vi "GUI.vi"() -> ()   [LabVIEW 2013]
uses:
  <vilib>/Instr/_visa.llb/VISA Configure Serial Port (Instr).vi
panel:
  out "Angle":u8[](array[numeric])
  out "Left":bool
  out "Right":bool
  out "read buffer":string
  in  "Stop":bool
  in  "Angle":string
  out "Error":errorcluster
  out "Arduino Data":string
  in  "Mode":bool
  in  "Baud Rate 2":u32=9600
  in  "Port 2":refnum<visa-resource-name>
  in  "Baud Rate":u32=9600
  in  "Port":refnum<visa-resource-name>
  out "Response 2":string
  in  "Command":string
  out "error out":errorcluster
  out "Numeric 12":i32
  in  "angle":i32
  in  "OK":bool
  in  "Commands":string(combo)
  out "error out 2":errorcluster
  in  "MODE":bool
  # "Arduino Interface"
  # "Encoder Interface"
  # "Text Mode"
  # "Button Mode"
  # "Select : ON : Text Mode , \n              OFF : ButtonMode"
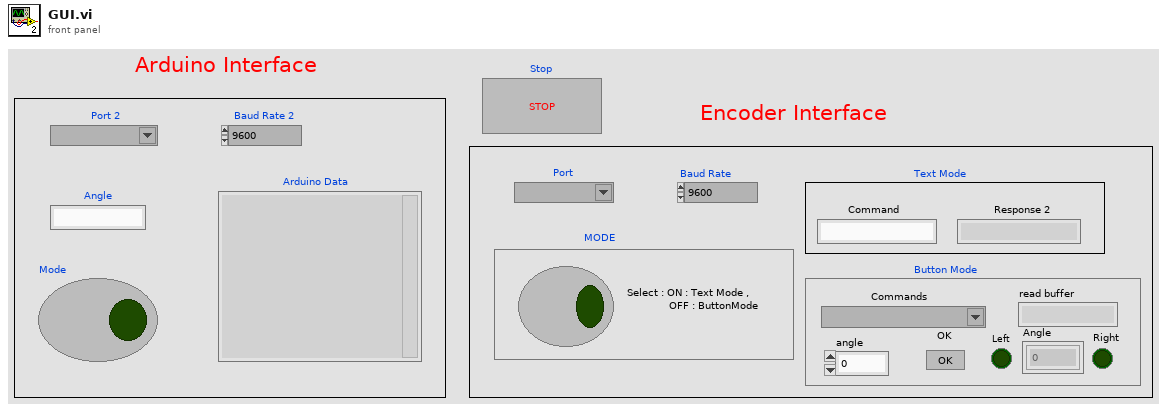
[diagram p1: front panel]
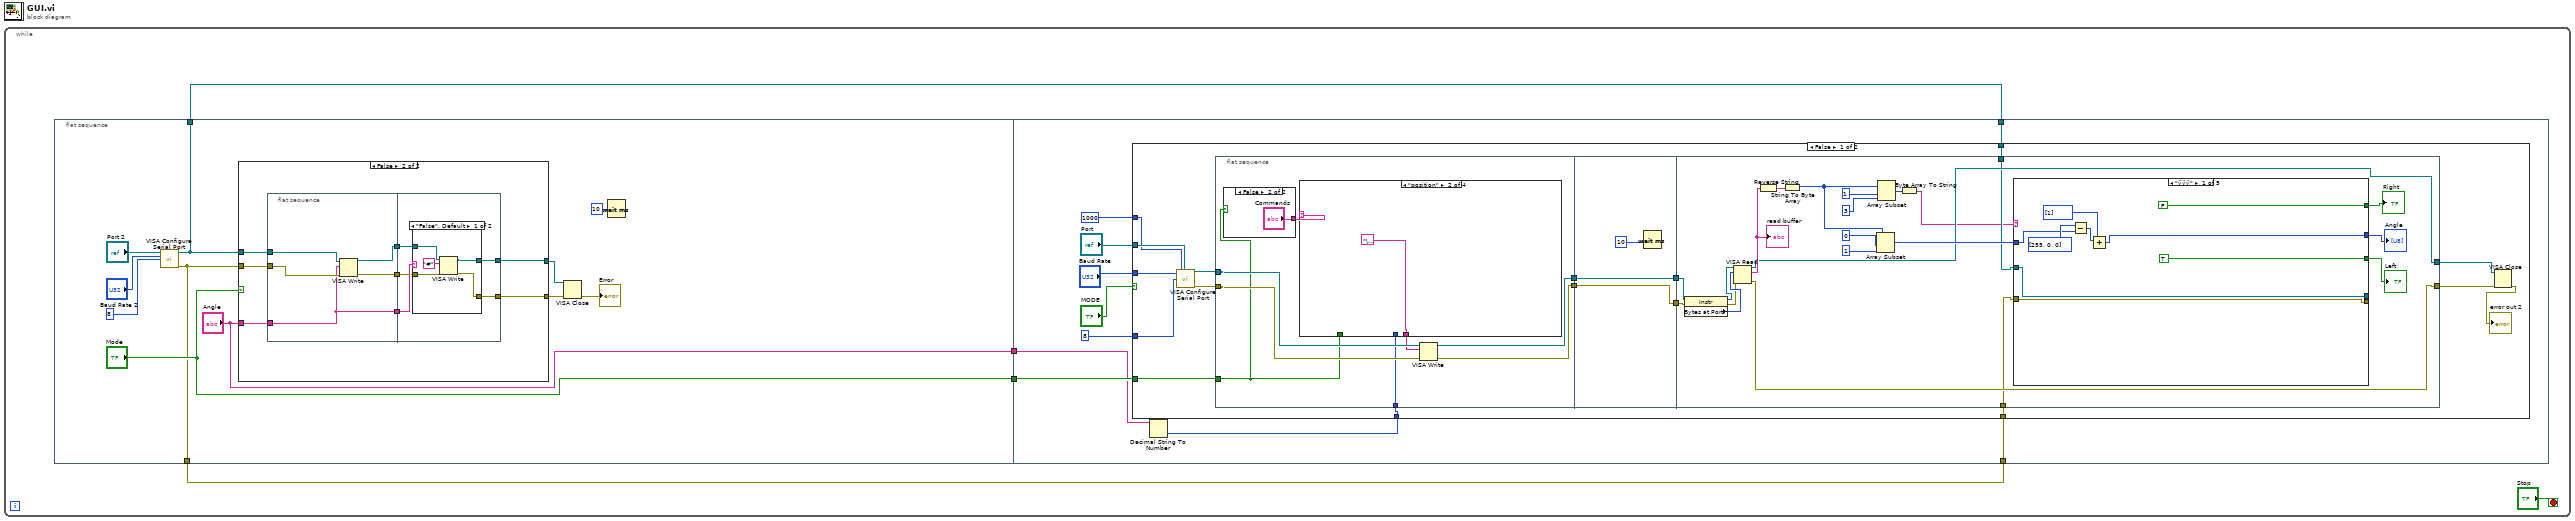
[diagram p0: block diagram]
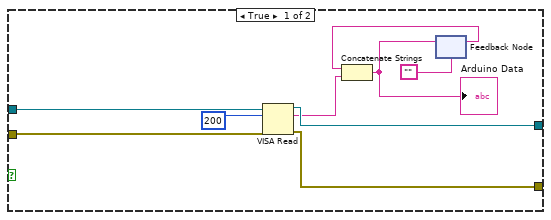
[diagram p2: hidden frame]
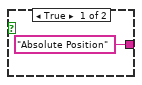
[diagram p4: hidden frame]
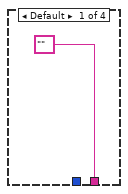
[diagram p5: hidden frame]
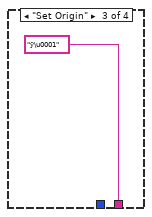
[diagram p6: hidden frame]
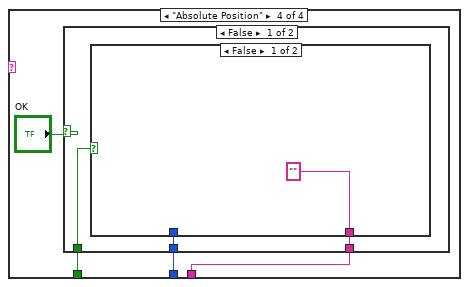
[diagram p7: hidden frame]
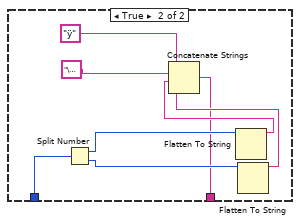
[diagram p8: hidden frame]
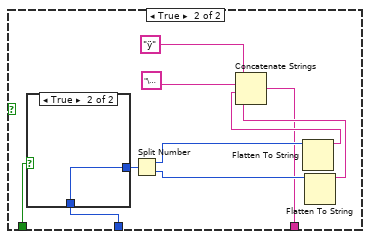
[diagram p9: hidden frame]
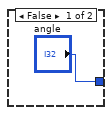
[diagram p10: hidden frame]
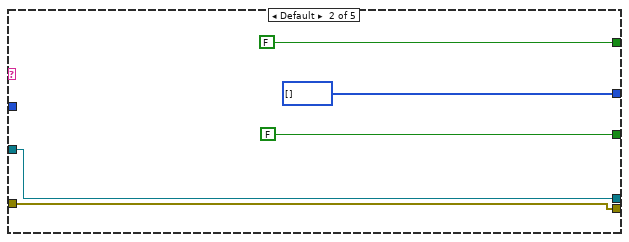
[diagram p11: hidden frame]
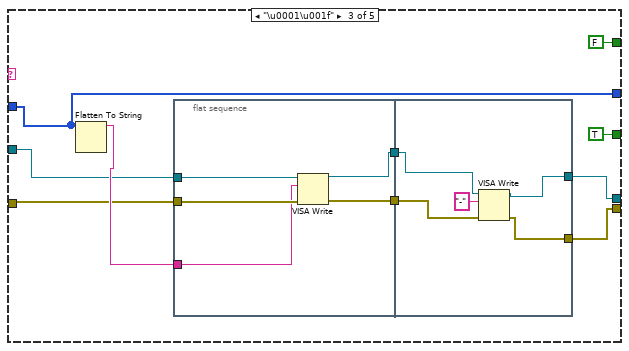
[diagram p12: hidden frame]
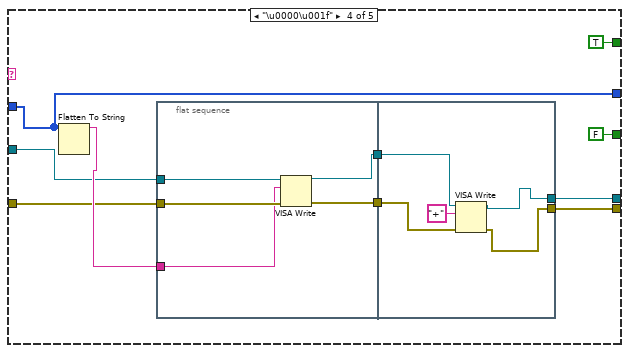
[diagram p13: hidden frame]
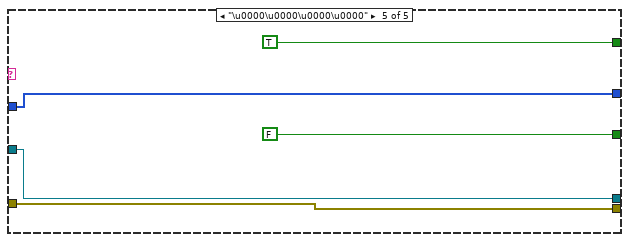
[diagram p14: hidden frame]
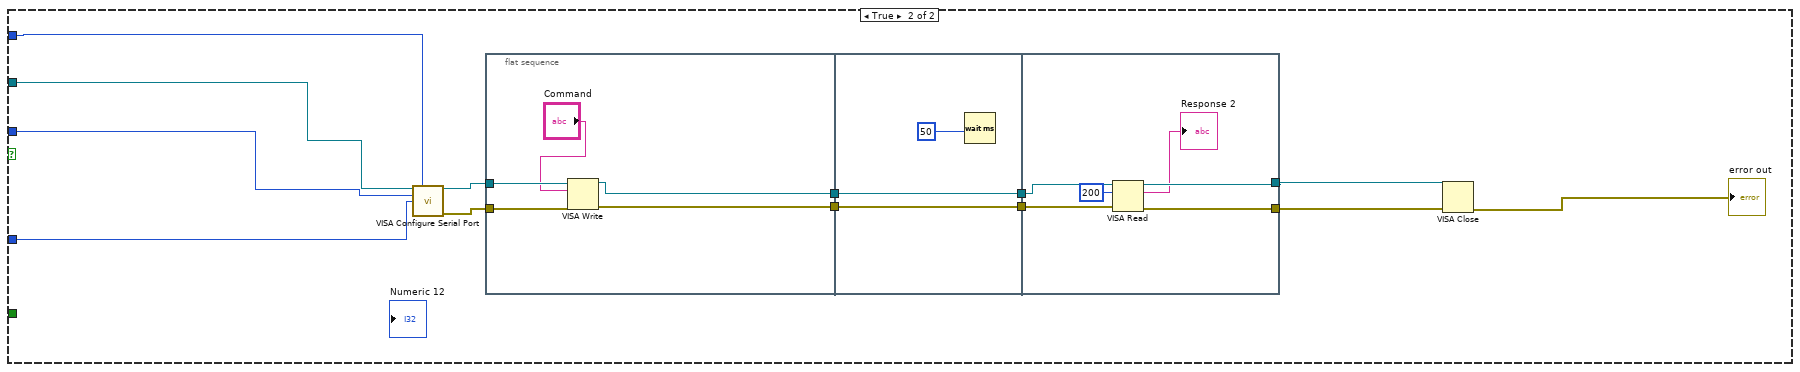
[diagram p15: hidden frame]
diagram:
  n1 = while {
    stop <- "Stop" stop-if-true
    n2 = flat-sequence {
      tunnel: ["Mode"] -> w5
      tunnel: ["Angle"] -> w4
      tunnel: [w7] -> w2
      tunnel: [w6] -> w1
      tunnel: w5 -> [w56]
      tunnel: w4 -> [w55]
      tunnel: w2 -> [w52]
      tunnel: w1 -> [w51]
      frame #0 {
        n3 = call-poly "VISA Configure Serial Port"("VISA resource name"="Port 2", "baud rate (9600)"="Baud Rate 2", "data bits (8)"=u16 8) -> ("VISA resource name out"=w7:refnum<visa-resource-name>, "error out"=w6:errorcluster)  [unwired: 11 in]
        n4 = case shown="False" "Mode" {
          tunnel: w7 -> [w23 w33]
          tunnel: [w24 w27] -> w15
          tunnel: [w25 w28] -> w16
          tunnel: w6 -> [w22 w32]
          tunnel: "Angle" -> [_ w26]
          frame True {
            n5 = VISA Read(VISA resource name=w23, byte count=u32 200, error in (no error)=w22) -> (VISA resource name out=w25:refnum<visa-resource-name>, read buffer=w20:string, error out=w24:errorcluster)  [unwired: 1 out]
            n6 = feedback #1("") -> (w19:string)
            n7 = Concatenate Strings(w19, w20) -> (w18:string)
            "Arduino Data" <- w18
            n8 = feedback-in #1(w18) -> ()
          }
          frame False {
            n9 = flat-sequence {
              tunnel: w33 -> [w38]
              tunnel: w32 -> [w37]
              tunnel: [w34] -> w31
              tunnel: [w36] -> w30
              tunnel: [w35] -> w29
              tunnel: w26 -> [w34]
              tunnel: w31 -> [w43]
              tunnel: w30 -> [w42]
              tunnel: w29 -> [w41]
              tunnel: [w40] -> w28
              tunnel: [w39] -> w27
              frame #0 {
                n10 = VISA Write(VISA resource name=w38, write buffer=w34, error in (no error)=w37) -> (VISA resource name out=w36:refnum<visa-resource-name>, error out=w35:errorcluster)  [unwired: 1 out]
              }
              frame #1 {
                n11 = case shown="\"False\", Default" w43 {
                  tunnel: w42 -> [w47 w50]
                  tunnel: w41 -> [w46 w49]
                  tunnel: [w45 w50] -> w40
                  tunnel: [w44 w49] -> w39
                  frame "False", Default {
                    n12 = VISA Write(VISA resource name=w47, write buffer="#", error in (no error)=w46) -> (VISA resource name out=w45:refnum<visa-resource-name>, error out=w44:errorcluster)  [unwired: 1 out]
                  }
                  frame "" {
                  }
                }
              }
            }
          }
        }
        n13 = VISA Close(VISA resource name=w16, error in (no error)=w15) -> (error out=→"Error":errorcluster)
        n14 = Wait (ms)(milliseconds to wait=u32 10) -> ()  [unwired: 1 out]
      }
      frame #1 {
        n15 = Decimal String To Number(string=w55) -> (number=w53:i32)  [unwired: 2 in, 1 out]
        n16 = case shown="False" "MODE" {
          tunnel: u32 1000 ("timeout (10sec)") -> [w65 w206]
          tunnel: "Port" -> [w71 w205]
          tunnel: "Baud Rate" -> [w70 w204]
          tunnel: u16 8 ("data bits (8)") -> [w67 w203]
          tunnel: w56 -> [w69 _]
          tunnel: w53 -> [w66 _]
          tunnel: w52 -> [w62 _]
          tunnel: w51 -> [w61 _]
          frame False {
            n17 = call-poly "VISA Configure Serial Port"("VISA resource name"=w71, "timeout (10sec)"=w65, "baud rate (9600)"=w70, "data bits (8)"=w67) -> ("VISA resource name out"=w75:refnum<visa-resource-name>, "error out"=w74:errorcluster)  [unwired: 10 in]
            n18 = flat-sequence {
              tunnel: [w84] -> w77
              tunnel: w75 -> [w83]
              tunnel: w74 -> [w82]
              tunnel: [w85] -> w73
              tunnel: w69 -> [w79]
              tunnel: w66 -> [w78]
              tunnel: [w120] -> w76
              tunnel: w77 -> [w119]
              tunnel: w73 -> [w120]
              tunnel: [w119] -> w72
              tunnel: w76 -> [w136]
              tunnel: w72 -> [w142]
              tunnel: [w126] -> w64
              tunnel: [w125] -> w63
              tunnel: w62 -> [w124]
              tunnel: w61 -> [w123]
              frame #0 {
                n19 = case shown="False" w79 {
                  tunnel: ["Absolute Position" ("Commands") "Commands"] -> w81
                  frame True {
                  }
                  frame False {
                  }
                }
                n20 = case shown="\"position\"" w81 {
                  tunnel: ["" "\u001f" "ÿ\u0001" w91] -> w80
                  tunnel: w79 -> [_ _ _ w93]
                  tunnel: w78 -> [_ _ _ w92]
                  frame Default {
                  }
                  frame "position" {
                  }
                  frame "Set Origin" {
                  }
                  frame "Absolute Position" {
                    n21 = case shown="False" "OK" {
                      tunnel: w93 -> [w97 w109]
                      tunnel: w92 -> [w96 w107]
                      tunnel: [w95 w108] -> w91
                      frame False {
                        n22 = case shown="False" w97 {
                          tunnel: w96 -> [_ w100]
                          tunnel: ["" w99] -> w95
                          frame False {
                          }
                          frame True {
                            n23 = Split Number(x=w100) -> (hi(x)=w102:u16, lo(x)=w101:u16)
                            n24 = Flatten To String(anything=w102) -> (data string=w104:string)  [unwired: 3 in, 2 out]
                            n25 = Flatten To String(anything=w101) -> (data string=w103:string)  [unwired: 3 in, 2 out]
                            n26 = Concatenate Strings("ÿ" ("string"), "\u0002" ("string"), w104, w103) -> (w99:string)
                          }
                        }
                      }
                      frame True {
                        n27 = case shown="True" w109 {
                          tunnel: w107 -> [_ w118]
                          tunnel: ["angle" w118] -> w110
                          frame False {
                          }
                          frame True {
                          }
                        }
                        n28 = Split Number(x=w110) -> (hi(x)=w112:u16, lo(x)=w111:u16)
                        n29 = Flatten To String(anything=w112) -> (data string=w114:string)  [unwired: 3 in, 2 out]
                        n30 = Flatten To String(anything=w111) -> (data string=w113:string)  [unwired: 3 in, 2 out]
                        n31 = Concatenate Strings("ÿ" ("string"), "\u0002" ("string"), w114, w113) -> (w108:string)
                      }
                    }
                  }
                }
                n32 = VISA Write(VISA resource name=w83, write buffer=w80, error in (no error)=w82) -> (VISA resource name out=w85:refnum<visa-resource-name>, error out=w84:errorcluster)  [unwired: 1 out]
              }
              frame #1 {
                n33 = Wait (ms)(milliseconds to wait=u32 10) -> ()  [unwired: 1 out]
              }
              frame #2 {
                n34 = property class="Instr"(reference=w136, error in=w142) -> (reference out=w135:refnum<visa-resource-name>, error out=w141:errorcluster, "Bytes at Port"=w143:u32)
                n35 = VISA Read(VISA resource name=w135, byte count=w143, error in (no error)=w141) -> (VISA resource name out=w126:refnum<visa-resource-name>, read buffer=w138:string, error out=w125:errorcluster)  [unwired: 1 out]
                "read buffer" <- w138
                n36 = Reverse String(1:w138) -> (0:w134:string)
                n37 = String To Byte Array(string=w134) -> (unsigned byte array=w140:u8[])
                n38 = Array Subset(array=w140, index=0, length=1) -> (w127:u8[])
                n39 = Array Subset(array=w140, index=1, length=3) -> (w137:u8[])
                n40 = Byte Array To String(unsigned byte array=w137) -> (string=w122:string)
                n41 = case shown="\"ÿÿÿ\"" w122 {
                  tunnel: [w149 u8[] [] w158 w178 w198] -> w129
                  tunnel: [TRUE ("Boolean") FALSE ("Boolean") TRUE ("Boolean") FALSE ("Boolean") FALSE ("Boolean")] -> w128
                  tunnel: [FALSE ("Boolean") FALSE ("Boolean") FALSE ("Boolean") TRUE ("Boolean") TRUE ("Boolean")] -> w130
                  tunnel: w123 -> [w146 w154 w161 w182 w200]
                  tunnel: [w145 w153 w160 w181 w199] -> _
                  tunnel: [w146 w154 w159 w180 w200] -> _
                  tunnel: w124 -> [w145 w153 w162 w179 w199]
                  tunnel: w127 -> [w144 _ w158 w178 w198]
                  frame "ÿÿÿ" {
                    n42 = Subtract(x=u8[] [255, 0, 0] ("y"), y=w144) -> (x-y=w152:u8[])
                    n43 = Add(x=w152, y=u8[] [1]) -> (x+y=w149:u8[])
                  }
                  frame Default {
                  }
                  frame "\u0001\u001f" {
                    n44 = Flatten To String(anything=w158) -> (data string=w163:string)  [unwired: 3 in, 2 out]
                    n45 = flat-sequence {
                      tunnel: [w172] -> w165
                      tunnel: [w171] -> w164
                      tunnel: w162 -> [w170]
                      tunnel: w161 -> [w169]
                      tunnel: w163 -> [w168]
                      tunnel: w165 -> [w176]
                      tunnel: w164 -> [w175]
                      tunnel: [w174] -> w160
                      tunnel: [w173] -> w159
                      frame #0 {
                        n46 = VISA Write(VISA resource name=w170, write buffer=w168, error in (no error)=w169) -> (VISA resource name out=w172:refnum<visa-resource-name>, error out=w171:errorcluster)  [unwired: 1 out]
                      }
                      frame #1 {
                        n47 = VISA Write(VISA resource name=w176, write buffer="-", error in (no error)=w175) -> (VISA resource name out=w174:refnum<visa-resource-name>, error out=w173:errorcluster)  [unwired: 1 out]
                      }
                    }
                  }
                  frame "\u0000\u001f" {
                    n48 = Flatten To String(anything=w178) -> (data string=w183:string)  [unwired: 3 in, 2 out]
                    n49 = flat-sequence {
                      tunnel: [w192] -> w185
                      tunnel: [w191] -> w184
                      tunnel: w179 -> [w190]
                      tunnel: w182 -> [w189]
                      tunnel: w183 -> [w188]
                      tunnel: w185 -> [w195]
                      tunnel: w184 -> [w196]
                      tunnel: [w194] -> w181
                      tunnel: [w193] -> w180
                      frame #0 {
                        n50 = VISA Write(VISA resource name=w190, write buffer=w188, error in (no error)=w189) -> (VISA resource name out=w192:refnum<visa-resource-name>, error out=w191:errorcluster)  [unwired: 1 out]
                      }
                      frame #1 {
                        n51 = VISA Write(VISA resource name=w195, write buffer="+", error in (no error)=w196) -> (VISA resource name out=w194:refnum<visa-resource-name>, error out=w193:errorcluster)  [unwired: 1 out]
                      }
                    }
                  }
                  frame "\u0000\u0000\u0000\u0000" {
                  }
                }
                "Left" <- w128
                "Right" <- w130
                "Angle" <- w129
              }
            }
            n52 = VISA Close(VISA resource name=w64, error in (no error)=w63) -> (error out=→"error out 2":errorcluster)
          }
          frame True {
            n53 = call-poly "VISA Configure Serial Port"("VISA resource name"=w205, "timeout (10sec)"=w206, "baud rate (9600)"=w204, "data bits (8)"=w203) -> ("VISA resource name out"=w211:refnum<visa-resource-name>, "error out"=w210:errorcluster)  [unwired: 10 in]
            n54 = flat-sequence {
              tunnel: w211 -> [w218]
              tunnel: w210 -> [w220]
              tunnel: [w217] -> w215
              tunnel: [w219] -> w214
              tunnel: [w222] -> w213
              tunnel: w215 -> [w222]
              tunnel: [w221] -> w212
              tunnel: w214 -> [w221]
              tunnel: w213 -> [w229]
              tunnel: w212 -> [w228]
              tunnel: [w227] -> w208
              tunnel: [w226] -> w209
              frame #0 {
                n55 = VISA Write(VISA resource name=w218, write buffer="Command", error in (no error)=w220) -> (VISA resource name out=w217:refnum<visa-resource-name>, error out=w219:errorcluster)  [unwired: 1 out]
              }
              frame #1 {
                n56 = Wait (ms)(milliseconds to wait=u32 50) -> ()  [unwired: 1 out]
              }
              frame #2 {
                n57 = VISA Read(VISA resource name=w229, byte count=u32 200, error in (no error)=w228) -> (VISA resource name out=w226:refnum<visa-resource-name>, read buffer=→"Response 2":string, error out=w227:errorcluster)  [unwired: 1 out]
              }
            }
            n58 = VISA Close(VISA resource name=w209, error in (no error)=w208) -> (error out=→"error out":errorcluster)
          }
        }
      }
    }
  }
